vi "Write layout.vi"(8 "error in (no error)":errorcluster, 10 "Lumberjack.lvlib:Layout.lvclass":refnum<class "Layout.lvclass">, 11 "ConsoleAppender in":refnum<class "ConsoleAppender.lvclass">) -> (0 "error out":errorcluster, 3 "ConsoleAppender out":refnum<class "ConsoleAppender.lvclass">)   [LabVIEW 2026, in "Lumberjack.lvlib" / "ConsoleAppender.lvclass"]
uses:
  ConsoleAppender.lvclass
  Layouts/Layout.lvclass/Layout.lvclass
  ConsoleAppender.lvclass/ConsoleAppender.ctl
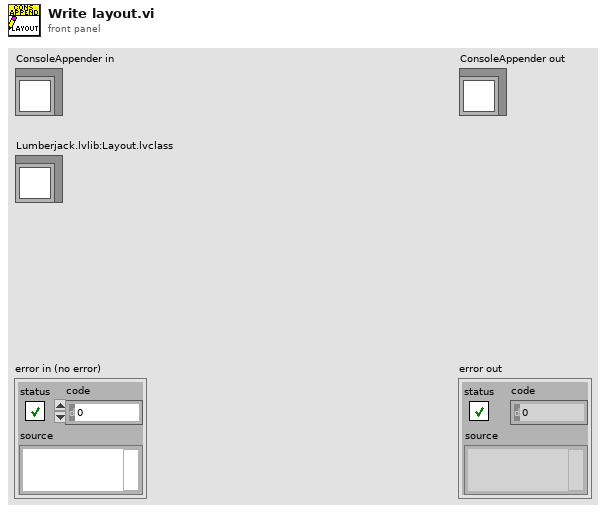
[diagram p1: front panel]
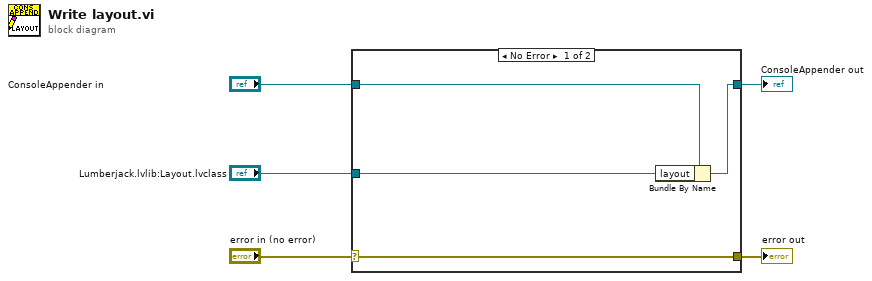
[diagram p0: block diagram]
diagram:
  n1 = case shown="No Error" "error in (no error)" {
    selector: "error in (no error)" -> [w9 w10]
    tunnel: [w9 w10] -> w4
    tunnel: [w7 w11] -> w2
    tunnel: "ConsoleAppender in" -> [w8 w11]
    tunnel: "Lumberjack.lvlib:Layout.lvclass" -> [w6 _]
    frame No Error {
      n2 = Bundle By Name(cluster=w8, "layout"=w6) -> (w7:refnum<class "ConsoleAppender.lvclass">)
    }
    frame Error {
    }
  }
  "error out" <- w4
  "ConsoleAppender out" <- w2
